vi "Display on Menu.vi"(7 "Menu Tag":string="Select Display", 8 "error in":errorcluster, 9 "Display information":T1, 10 "Active Display":u16, 11 "Menu Ref":refnum<k9>) -> (0 "error out":errorcluster, 3 "Menu Ref":refnum<k9>)   [LabVIEW 2014]
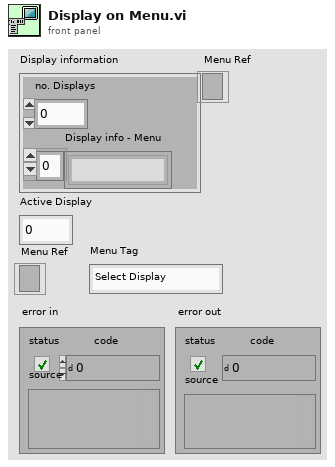
[diagram p1: front panel]
types:
  T1 = cluster{"no. Displays":i32, "Display info - Menu":string[]}
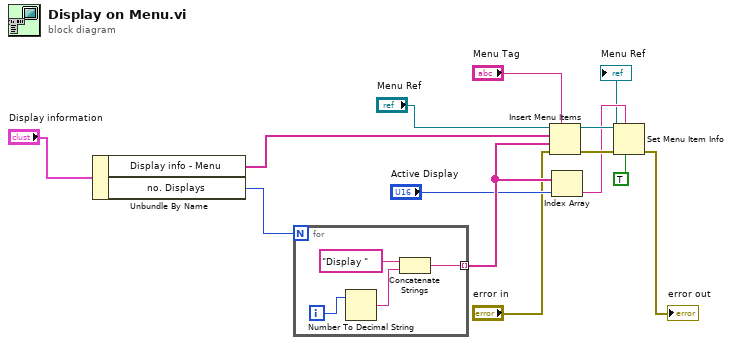
[diagram p0: block diagram]
diagram:
  n1 = Unbundle By Name("Display information") -> ("Display info - Menu"=w5:string[], "no. Displays"=w12:i32)
  n2 = for {
    N: w12 -> [_]
    tunnel: [w14] -> w4 mode=indexing
    i -> [w16]
    n3 = Number To Decimal String(number=w16) -> (decimal integer string=w15:string)  [unwired: 1 in]
    n4 = Concatenate Strings("Display ", w15) -> (w14:string)
  }
  n5 = Insert Menu Items(5:"Menu Tag", 6:"error in", 7:w4, 8:w5, 9:"Menu Ref") -> (0:w11:errorcluster, 3:w10:refnum<k9>)  [unwired: 1 in, 1 out]
  n6 = Index Array(array=w4, index="Active Display") -> (element=w8:string)
  n7 = Set Menu Item Info(6:TRUE ("checked"), 7:w8, 8:w11, 11:w10) -> (0:→"error out":errorcluster)  [unwired: 3 in, 1 out]
  "Menu Ref" <- "Menu Ref"
